vi "lvlibp-test-Main.vi"(8 "error in (no error)":errorcluster, 10 "name":string="numeric", 11 "TagDB":T1) -> (0 "error out":errorcluster, 2 "Value":i32)   [LabVIEW 2017, in "tagdb-tester.lvlib"]
uses:
  tagdb-tester.lvlib
  src/TagDB/Typedef/TagDB.ctl
  src/TagDB/_Support/Error/_Build Error Cluster.vi
  src/TagDB/TagDB.lvlib
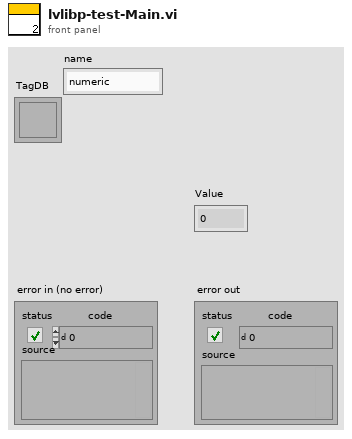
[diagram p1: front panel]
types:
  T1 = typedef "TagDB.lvlib/TagDB.ctl" = refnum<k1>
  T2 = typedef "TagDB.lvlib/tagdb-data.ctl" = cluster{"tag-map":variant, "timestamp-map":variant, "namecacher-map":variant, "DataTypeCacher-map":variant, "Tag Adding Lock?":bool, "Global Change Timestamp":timestamp, "Item Change Timestamp":timestamp, "name":string, "Global Change Flag":u64, "Item Change Flag":u64}
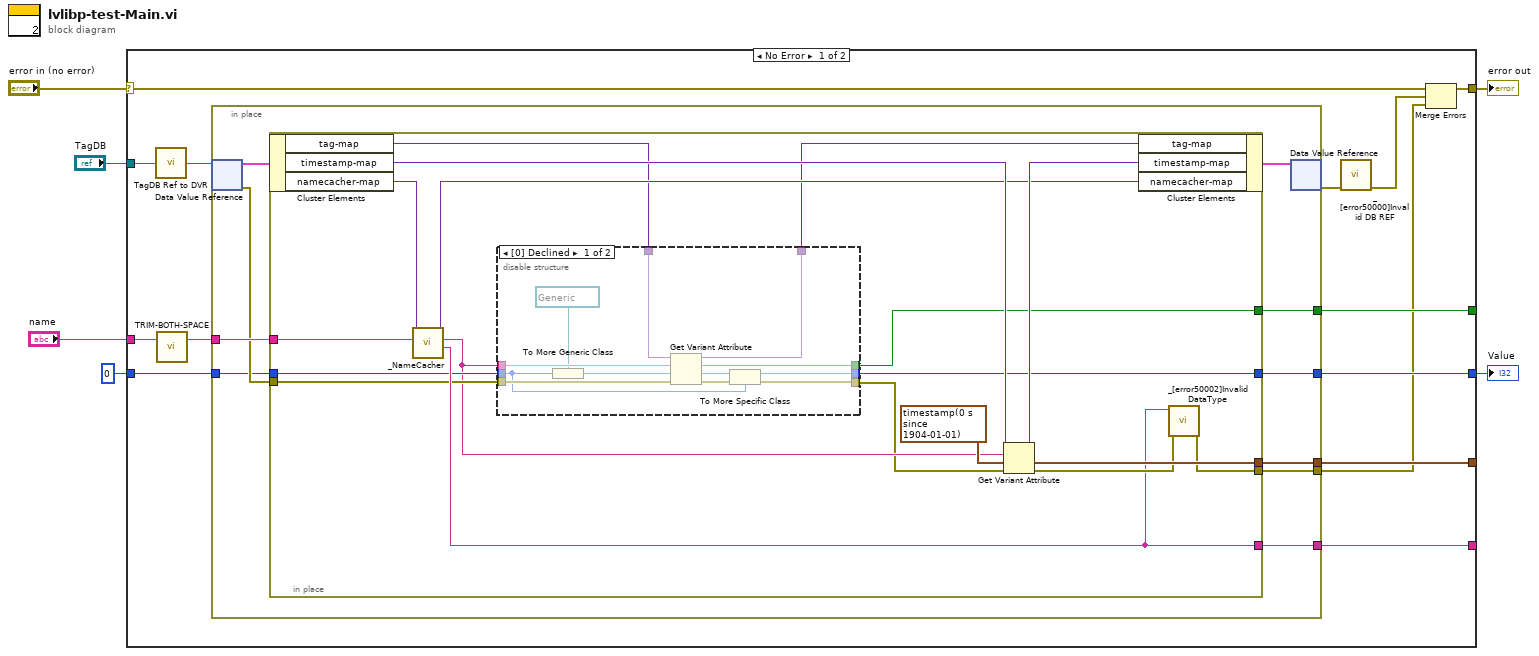
[diagram p0: block diagram]
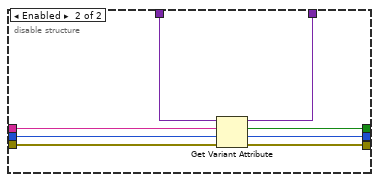
[diagram p2: hidden frame]
diagram:
  n1 = case shown="No Error" "error in (no error)" {
    selector: "error in (no error)" -> [w19 w70]
    tunnel: [w20 w70] -> w2
    tunnel: "name" -> [w10 _]
    tunnel: "TagDB" -> [w17 _]
    tunnel: [w16 w69] -> w3
    tunnel: 0 -> [w15 w69]
    tunnel: [w14 _] -> _
    tunnel: [w12 _] -> _
    tunnel: [w9 _] -> _
    frame No Error {
      n2 = call "TagDB Ref to DVR.vi"("TagDB"=w17) -> ("DVR"=w13:refnum<data-value>)  [unwired: 4 in]
      n3 = call "TRIM-BOTH-SPACE.vi"("name in"=w10) -> ("name out"=w7:string)  [unwired: 2 in]
      n4 = in-place "In Place Element Structure" {
        in-place-border: [w22] -> w16
        in-place-border: w15 -> [w23]
        in-place-border: [w21] -> w14
        in-place-border: [w30] -> w12
        in-place-border: [w29] -> w11
        in-place-border: w7 -> [w28]
        in-place-border: [w27] -> w9
        n5 = in-place-dvr #1(w13) -> (w26:T2, w24:errorcluster)
        n6 = in-place {
          in-place-border: [w48] -> w30
          in-place-border: [w41] -> w29
          in-place-border: w28 -> [w47]
          in-place-border: [w40] -> w27
          in-place-border: w24 -> [w38]
          in-place-border: w23 -> [w37]
          in-place-border: [w33] -> w22
          in-place-border: [w32] -> w21
          n7 = in-place-cluster #2(w26) -> ("tag-map"=w35:variant, "timestamp-map"=w46:variant, "namecacher-map"=w45:variant)
          n8 = call "_NameCacher.vi"("key"=w47, "cacher"=w45) -> ("Raw name"=w40:string, "Key in lower case"=w36:string, "cacher out"=w43:variant)  [unwired: 7 in]
          n9 = disable-structure shown="[0] Declined" {
            disable-tunnel: w38 -> [w60 w68]
            disable-tunnel: w37 -> [w49 w67]
            disable-tunnel: w36 -> [w59 w66]
            disable-tunnel: w35 -> [w58 w65]
            disable-tunnel: [w50 w64] -> w34
            disable-tunnel: [w52 w63] -> w33
            disable-tunnel: [w56 w62] -> w32
            disable-tunnel: [w55 w61] -> w31
            frame Disabled {
              n10 = To More Generic Class(target class=refnum<vi> refnum ("value"), reference=w49) -> (generic class reference=w53:refnum<vi>)
              n11 = Get Variant Attribute(Variant=w58, name=w59, default value (empty Variant)=w53, error in=w60) -> (duplicate Variant=w55:variant, found=w56:bool, value=w57:refnum<vi>, error out=w51:errorcluster)
              n12 = To More Specific Class(target class=w49, reference=w57, error in=w51) -> (specific class reference=w52:refnum<vi>, error out=w50:errorcluster)
            }
            frame Enabled {
              n13 = Get Variant Attribute(Variant=w65, name=w66, default value (empty Variant)=w67, error in=w68) -> (duplicate Variant=w61:variant, found=w62:bool, value=w63:i32, error out=w64:errorcluster)
            }
          }
          n14 = Get Variant Attribute(Variant=w46, name=w36, default value (empty Variant)=timestamp(0 s since 1904-01-01) ("Time Stamp"), error in=w34) -> (duplicate Variant=w44:variant, value=w48:timestamp, error out=w42:errorcluster)  [unwired: 1 out]
          n15 = in-place-cluster #2("tag-map"=w31, "timestamp-map"=w44, "namecacher-map"=w43) -> (w25:T2)
          n16 = call "_[error50002]Invalid DataType.vi"("error in (no error)"=w42, "string"=w40) -> ("error out"=w41:errorcluster)  [unwired: 9 in]
        }
        n17 = in-place-dvr #1(w25) -> (w18:errorcluster)  [unwired: 1 out]
      }
      n18 = call "_[error50000]Invalid DB REF.vi"("error in (no error)"=w18) -> ("error out"=w8:errorcluster)  [unwired: 10 in]
      n19 = Merge Errors(w19, w8, w11) -> (w20:errorcluster)
    }
    frame Error {
    }
  }
  "Value" <- w3
  "error out" <- w2
